vi "StringList.Add Items.vi"(8 "error in (no error)":errorcluster, 9 "New Items":string[](array[string]), 10 "New Item":string, 11 "StringList in":refnum<class "StringList.lvclass">) -> (0 "error out":errorcluster, 2 "Items Out":string[](array[string]), 3 "StringList out":refnum<class "StringList.lvclass">)   [LabVIEW 2024, in "StringList.lvclass"]
uses:
  StringList.lvclass
  StringList.lvclass/StringList.ctl
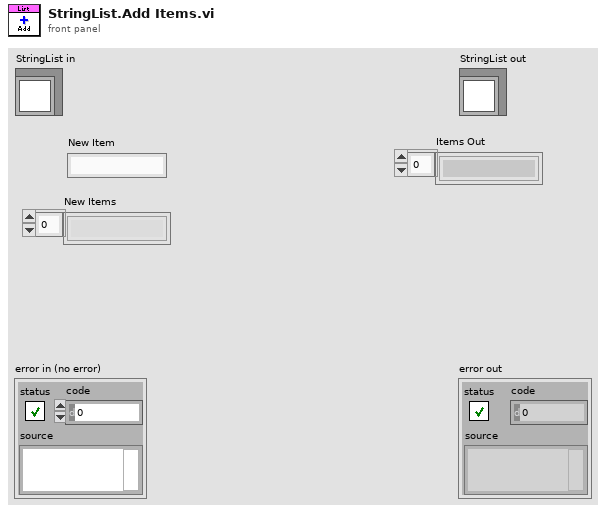
[diagram p1: front panel]
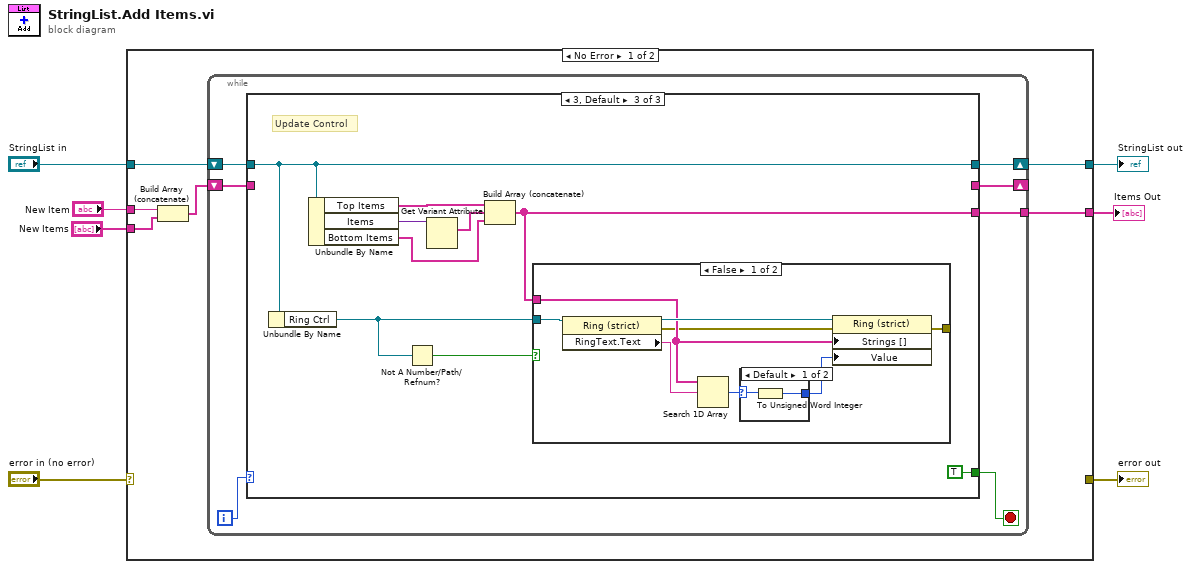
[diagram p0: block diagram]
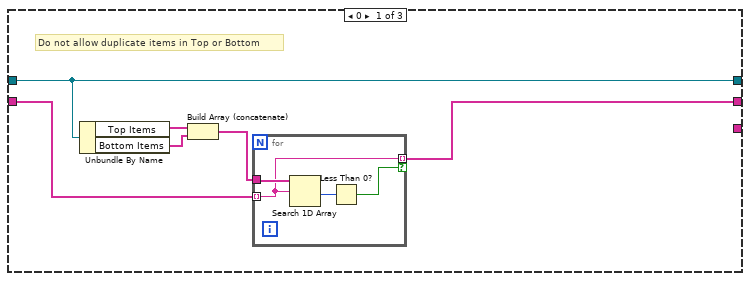
[diagram p2: hidden frame]
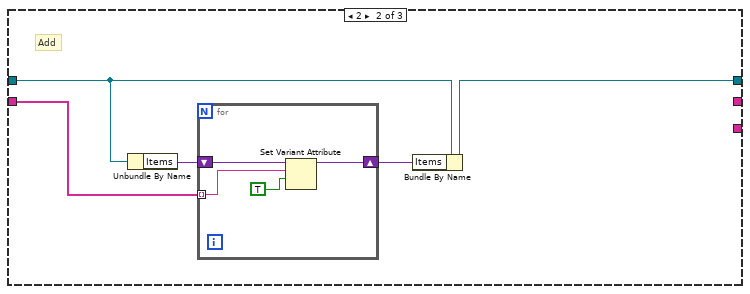
[diagram p3: hidden frame]
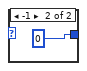
[diagram p4: hidden frame]
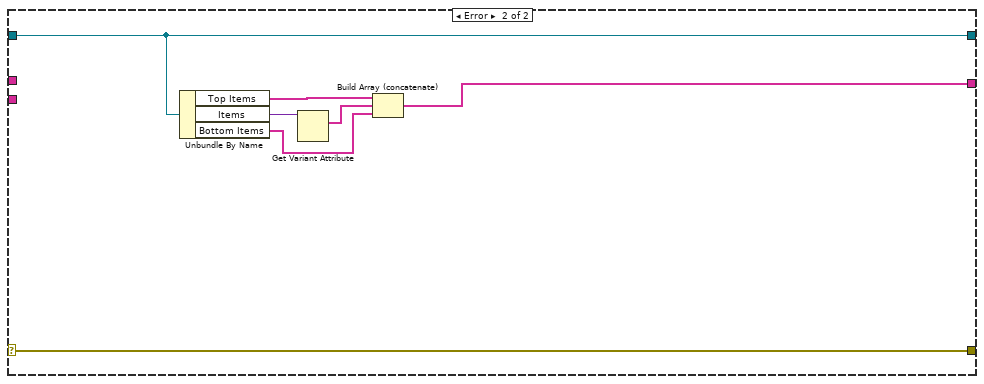
[diagram p6: hidden frame]
diagram:
  n1 = case shown="No Error" "error in (no error)" {
    selector: "error in (no error)" -> [_ w66]
    tunnel: [_ w66] -> w6
    tunnel: [w13 w61] -> w4
    tunnel: "StringList in" -> [w12 w61]
    tunnel: "New Item" -> [w11 _]
    tunnel: "New Items" -> [w10 _]
    tunnel: [w8 w60] -> w1
    frame No Error {
      n2 = Build Array (concatenate)(w11, w10) -> (w9:string[])
      n3 = while {
        shift-right: [w19] -> w13
        shift-left: w12 -> [w18]
        shift-right: [w15] -> _
        shift-left: w9 -> [w20]
        tunnel: [w14] -> w8
        i -> [w17]
        stop <- w16 stop-if-true
        n4 = case shown="3, Default" w17 {
          tunnel: w20 -> [w26 w32 _]
          tunnel: [w22 w35 w48] -> w19
          tunnel: w18 -> [w22 w34 w48]
          tunnel: [_ _ TRUE] -> w16
          tunnel: [w21 _ _] -> w15
          tunnel: [_ _ w42] -> w14
          frame 0 {
            # "Do not allow duplicate items in Top or Bottom"
            n5 = Unbundle By Name(w22) -> ("Top Items"=w25:string[], "Bottom Items"=w24:string[])
            n6 = Build Array (concatenate)(w25, w24) -> (w23:string[])
            n7 = for {
              tunnel: w26 -> [w28] mode=indexing
              tunnel: w23 -> [w30]
              tunnel: [w28] -> w21 mode=indexing if=w27
              n8 = Search 1D Array(1D array=w30, element=w28) -> (index of element=w29:i32)  [unwired: 1 in]
              n9 = Less Than 0?(x=w29) -> (x < 0?=w27:bool)
            }
          }
          frame 2 {
            # "Add"
            n10 = Unbundle By Name(w34) -> ("Items"=w33:variant)
            n11 = for {
              tunnel: w32 -> [w38] mode=indexing
              shift-right: [w36] -> w31
              shift-left: w33 -> [w39]
              n12 = Set Variant Attribute(Variant=w39, name=w38, value=TRUE) -> (Variant out=w36:variant)  [unwired: 1 in, 2 out]
            }
            n13 = Bundle By Name(cluster=w34, "Items"=w31) -> (w35:refnum<class "StringList.lvclass">)
          }
          frame 3, Default {
            # "Update Control"
            n14 = Unbundle By Name(w48) -> ("Ring Ctrl"=w47:refnum<vi>)
            n15 = Unbundle By Name(w48) -> ("Top Items"=w46:string[], "Items"=w44:variant, "Bottom Items"=w45:string[])
            n16 = Not A Number/Path/Refnum?(number/path/refnum=w47) -> (NaN/Path/Refnum?=w40:bool)
            n17 = Get Variant Attribute(Variant=w44) -> (names=w43:string[])  [unwired: 3 in, 3 out]
            n18 = Build Array (concatenate)(w46, w43, w45) -> (w42:string[])
            n19 = case shown="False" w40 {
              tunnel: w47 -> [w56 _]
              tunnel: w42 -> [w54 _]
              tunnel: [w50 _] -> _
              frame False {
                n20 = property class="Ring (strict)"(reference=w56) -> (reference out=w55:refnum<vi>, error out=w49:errorcluster, "RingText.Text"=w53:string)  [unwired: 1 in]
                n21 = Search 1D Array(1D array=w54, element=w53) -> (index of element=w52:i32)  [unwired: 1 in]
                n22 = case shown="Default" w52 {
                  selector: w52 -> [w58 _]
                  tunnel: [w57 u16 0 ("Value")] -> w51
                  frame Default {
                    n23 = To Unsigned Word Integer(number=w58) -> (unsigned 16bit integer=w57:u16)
                  }
                  frame -1 {
                  }
                }
                n24 = property class="Ring (strict)"(reference=w55, error in=w49, "Strings []"=w54, "Value"=w51) -> (error out=w50:errorcluster)  [unwired: 1 out]
              }
              frame True {
              }
            }
          }
        }
      }
    }
    frame Error {
      n25 = Unbundle By Name(w61) -> ("Top Items"=w65:string[], "Items"=w63:variant, "Bottom Items"=w64:string[])
      n26 = Get Variant Attribute(Variant=w63) -> (names=w62:string[])  [unwired: 3 in, 3 out]
      n27 = Build Array (concatenate)(w65, w62, w64) -> (w60:string[])
    }
  }
  "error out" <- w6
  "StringList out" <- w4
  "Items Out" <- w1
